vi "Buffer (parameters) v1.00.vi"(0 "FilePath In":path=path "/DATA/Xing Wei Data/MyData.010", 1 "Read#":u8=10, 2 "Action":u8(ring)=1 items=["Read", "Write", "Initialize"], 7 "Field In":dbl format="%.2f", 11 "Temperature In":dbl=-1.0 format="%.2f", 12 "FilePath Buffer in":path[](array[path])=[path "/DATA/Labview Temporary Items"], 13 "Field Buffer in":dbl[](array[numeric])=[0.0] format="%.2f", 14 "Temperature Buffer in":dbl[](array[numeric])=[0.0] format="%.2f") -> (4 "FilePath out":path, 6 "Field Out":dbl format="%.2f", 8 "Temperature Out":dbl format="%.2f", 10 "Current Buffer Size":i32=11, 15 "Read Error":bool)   [LabVIEW 2024]
doc: "Write (FIFO) or retrieve (LIFO) data from the buffer.\n\nWhen write to the buffer, set the desired \"Buffer Size\" and run the VI several iterations. Notice that initially, the buffer grows to reach \"Buffer Size\" and then the input data flows from the last buffer element through to the zero element on each iteration (First In, First Out).\n\nWhen read from the buffer, set the Read# to the nth previous input data, i.e. counting reversely, with the most recent input counted as the 1st readout. If the input is out of current buffer size, an error is returned. (Last In, First Out)"
uses:
  Globals and TypeDefs/Global Varibal Control.vi
panel:
  out "Temperature Buffer":dbl[](array[numeric])=[-1.0, -1.0, -1.0, -1.0, -1.0, -1.0, -1.0, -1.0, -1.0, -1.0] format="%.2f"
  out "Field Buffer":dbl[](array[numeric]) format="%.2f"
  out "FilePath Buffer":path[](array[path])=[path "/DATA/Xing Wei Data/MyData.001", path "/DATA/Xing Wei Data/MyData.002", path "/DATA/Xing Wei Data/MyData.003", path "/DATA/Xing Wei Data/MyData.004", path "/DATA/Xing Wei Data/MyData.005", path "/DATA/Xing Wei Data/MyData.006", path "/DATA/Xing Wei Data/MyData.007", path "/DATA/Xing Wei Data/MyData.008", path "/DATA/Xing Wei Data/MyData.009", path "/DATA/Xing Wei Data/MyData.010"]
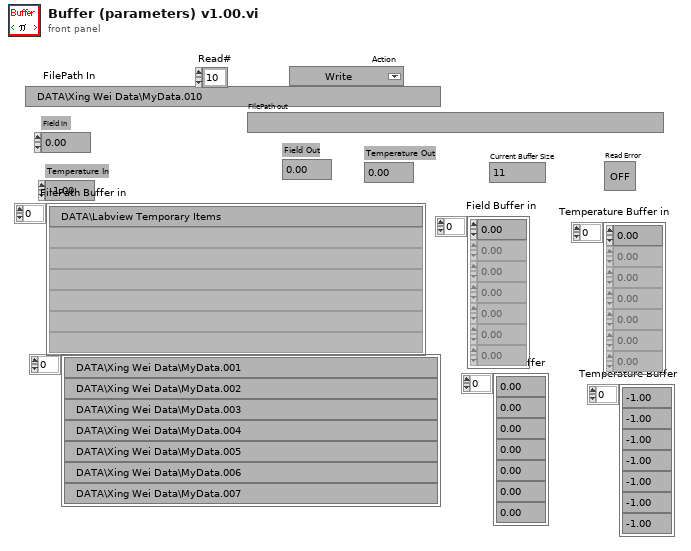
[diagram p1: front panel]
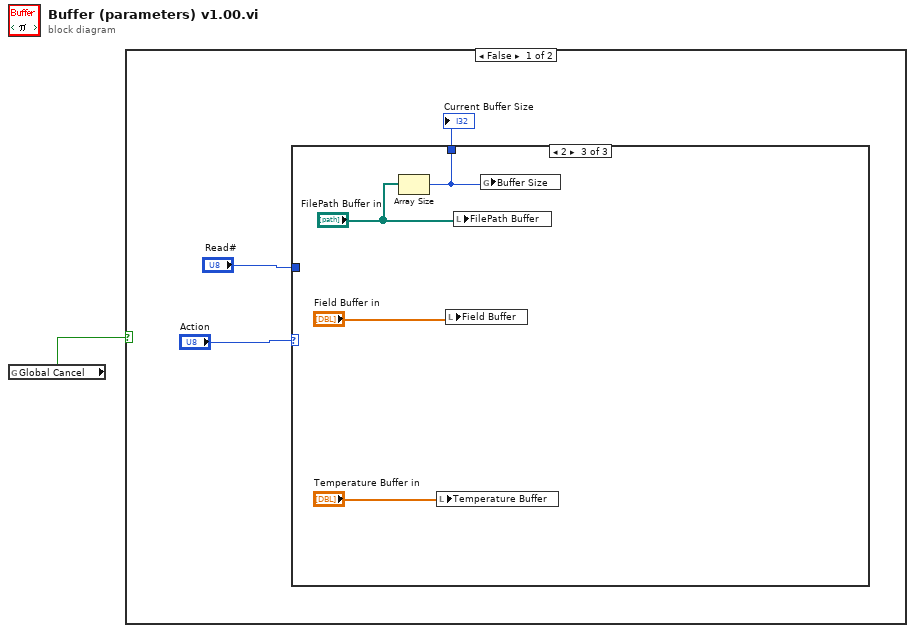
[diagram p0: block diagram]
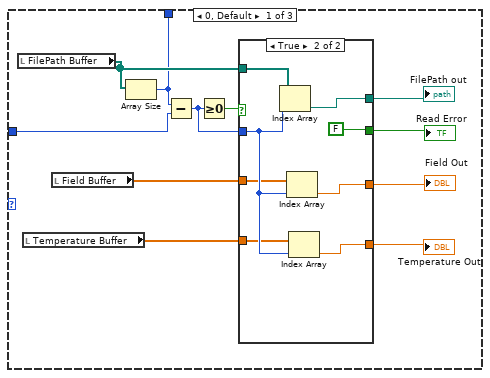
[diagram p2: hidden frame]
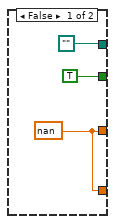
[diagram p3: hidden frame]
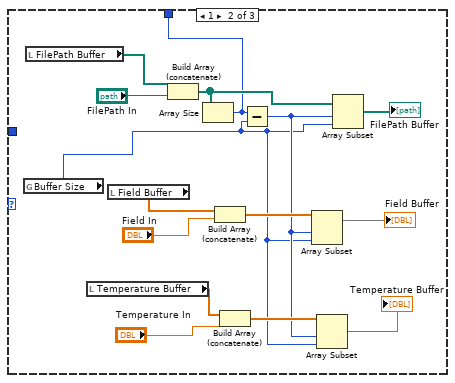
[diagram p4: hidden frame]
diagram:
  n1 = global read "Global Varibal Control.vi" "Global Cancel"() -> (w1:bool)
  n2 = case shown="False" w1 {
    frame False {
      n3 = case shown="2" "Action" {
        tunnel: "Read#" -> [w14 _ _]
        tunnel: [w11 w40 w42] -> w3
        frame 0, Default {
          n4 = local read "FilePath Buffer"() -> (w15:path[])
          n5 = local read "Temperature Buffer"() -> (w7:dbl[])
          n6 = local read "Field Buffer"() -> (w8:dbl[])
          n7 = Array Size(array=w15) -> (size(s)=w11:i32)
          n8 = Subtract(x=w11, y=w14) -> (x-y=w12:i32)
          n9 = Greater Or Equal To 0?(x=w12) -> (x >= 0?=w13:bool)
          n10 = case shown="True" w13 {
            tunnel: w15 -> [_ w26]
            tunnel: w12 -> [_ w23]
            tunnel: [path "" w25] -> w10
            tunnel: [TRUE FALSE] -> w9
            tunnel: w8 -> [_ w22]
            tunnel: w7 -> [_ w21]
            tunnel: [w16 w20] -> w6
            tunnel: [w16 w19] -> w5
            frame False {
              w16 = nan ("sqrt(x)")
            }
            frame True {
              n11 = Index Array(array=w26, index=w23) -> (element=w25:path)
              n12 = Index Array(array=w22, index=w23) -> (element=w20:dbl)
              n13 = Index Array(array=w21, index=w23) -> (element=w19:dbl)
            }
          }
          "FilePath out" <- w10
          "Read Error" <- w9
          "Field Out" <- w6
          "Temperature Out" <- w5
        }
        frame 1 {
          n14 = global read "Global Varibal Control.vi" "Buffer Size"() -> (w27:u8)
          n15 = local read "FilePath Buffer"() -> (w28:path[])
          n16 = local read "Temperature Buffer"() -> (w31:dbl[])
          n17 = local read "Field Buffer"() -> (w33:dbl[])
          n18 = Build Array (concatenate)(w28, "FilePath In") -> (w41:path[])
          n19 = Array Size(array=w41) -> (size(s)=w40:i32)
          n20 = Build Array (concatenate)(w33, "Field In") -> (w37:dbl[])
          n21 = Build Array (concatenate)(w31, "Temperature In") -> (w36:dbl[])
          n22 = Subtract(x=w40, y=w27) -> (x-y=w35:i32)
          n23 = Array Subset(array=w37, index=w35, length=w27) -> (→"Field Buffer":dbl[])
          n24 = Array Subset(array=w36, index=w35, length=w27) -> (→"Temperature Buffer":dbl[])
          n25 = Array Subset(array=w41, index=w35, length=w27) -> (→"FilePath Buffer":path[])
        }
        frame 2 {
          n26 = Array Size(array="FilePath Buffer in") -> (size(s)=w42:i32)
          n27 = local write "Temperature Buffer"("Temperature Buffer in") -> ()
          n28 = local write "Field Buffer"("Field Buffer in") -> ()
          n29 = local write "FilePath Buffer"("FilePath Buffer in") -> ()
          n30 = global write "Global Varibal Control.vi" "Buffer Size"(w42) -> ()
        }
      }
      "Current Buffer Size" <- w3
    }
    frame True {
    }
  }
